vi "ConfigFunction.vi"(8 "error in (no error)":errorcluster, 11 "NiPxi6733 in":refnum<class "NiPxi6733.lvclass">) -> (0 "error out":errorcluster, 3 "NiPxi6733 out":refnum<class "NiPxi6733.lvclass">)   [LabVIEW 2014, in "FgenPlugins.lvlib" / "NiPxi6733.lvclass"]
uses:
  NiPxi6733.lvclass
  FgenPluginBaseClass/FgenPluginsBase.lvclass/FgenPluginsBase.ctl
  NiPxi6733.lvclass/NiPxi6733.ctl
  FgenPluginBaseClass/Accessors/Read FunctionClass.vi
  Accessors/Read SampleRate.vi
  FgenPluginBaseClass/Accessors/Write FunctionClass.vi
  MemberClasses/FunctionBaseClass/FunctionBase.lvclass
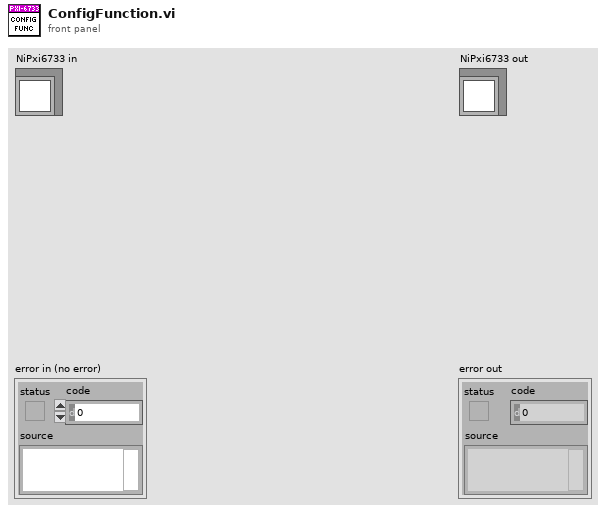
[diagram p1: front panel]
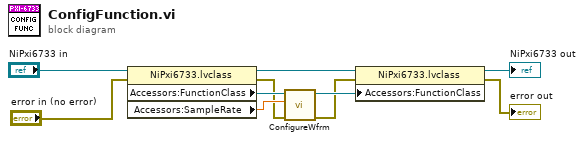
[diagram p0: block diagram]
diagram:
  n1 = property class="NiPxi6733.lvclass"(reference="NiPxi6733 in", error in="error in (no error)") -> (reference out=w4:refnum<class "NiPxi6733.lvclass">, error out=w6:errorcluster, "Accessors:FunctionClass"=w8:refnum<class "FunctionBase.lvclass">, "Accessors:SampleRate"=w7:dbl)
  n2 = call-dynamic "ConfigureWfrm.vi"("error in (no error)"=w6, "SampleRate"=w7, "FunctionBase in"=w8) -> ("error out"=w3:errorcluster, "FunctionBase out"=w5:refnum<class "FunctionBase.lvclass">)  [unwired: 7 in]
  n3 = property class="NiPxi6733.lvclass"(reference=w4, error in=w3, "Accessors:FunctionClass"=w5) -> (reference out=→"NiPxi6733 out":refnum<class "NiPxi6733.lvclass">, error out=→"error out":errorcluster)
